vi "ESPControl.vi"(0 "Motion Settings":T1={"No Motion?"=FALSE, "Motion System"=enum."NI 735x", "Motion Bd ID"=1, "Motion Profile"="SMAC1", "# Axis"=1, "Reverse Z axis?"=TRUE, "SMAC Axis"=0, "scan pair"=enum."y-(x) scan", "RT fps"=6.0, "Steps per mm"=[1000, 1000, 1000, 1000], "Motor Parameters"={"velocity ct/s"=[10000.0, 10000.0, 10000.0, 50000.0], "accel ct/s^2"=[50000.0, 50000.0, 50000.0, 200000.0]}, "One Way Scan"=FALSE, "Reverse One Way Scan"=FALSE, "Global Position (mm)"=[], "Plane"=0, "Distance between\nscan lines (um)"=0.0, "Distance between\nscan planes (um)"=0.0, "number of scan planes"=1, "Total steps in line"=0, "Xtra plane\ndistance  (um)"=100, "Xtra planes "=1, "Add Axis"=FALSE, "overshoot cts"=200, "BKPT Shift"=0, "Scan Start Time (ms)"=0, "ESP VISA"="GPIB::1::INSTR", "3rd Axis"=1, "GL Ref Out"=refnum, "Galil Address"=""} {"3rd Axis" items=["x", "y", "z", "w"]; "Xtra planes" min=1; "Xtra plane\ndistance  (um)" min=0; "Distance between\nscan planes (um)" format="%.2f"; "Distance between\nscan lines (um)" format="%.2f"; "SMAC Axis" items=["None"=0, "Axis 1"=1, "Axis 2"=2, "Axis 3"=3, "Axis 4"=4, "Axis 5"=5, "Axis 6"=6, "Axis 7"=7, "Axis 8"=8, "Vector Space 1"=17, "Vector Space 2"=18, "Vector Space 3"=19, "Vector Space 4"=20]; "Motion Bd ID" min=1 max=32 step=1}, 1 "# Axis":u16=2) -> (5 "VISA resource name out":refnum<visa-resource-name>="GPIB::1::INSTR", 6 "Motion Settings Out":T1={"No Motion?"=FALSE, "Motion System"=enum."NI 735x", "Motion Bd ID"=1, "Motion Profile"="SMAC1", "# Axis"=1, "Reverse Z axis?"=TRUE, "SMAC Axis"=0, "scan pair"=enum."y-(x) scan", "RT fps"=6.0, "Steps per mm"=[1000, 1000, 1000, 1000], "Motor Parameters"={"velocity ct/s"=[10000.0, 10000.0, 10000.0, 50000.0], "accel ct/s^2"=[50000.0, 50000.0, 50000.0, 200000.0]}, "One Way Scan"=FALSE, "Reverse One Way Scan"=FALSE, "Global Position (mm)"=[], "Plane"=0, "Distance between\nscan lines (um)"=0.0, "Distance between\nscan planes (um)"=0.0, "number of scan planes"=1, "Total steps in line"=0, "Xtra plane\ndistance  (um)"=100, "Xtra planes "=1, "Add Axis"=FALSE, "overshoot cts"=200, "BKPT Shift"=0, "Scan Start Time (ms)"=0, "ESP VISA"="GPIB::1::INSTR", "3rd Axis"=1, "GL Ref Out"=refnum, "Galil Address"=""} {"3rd Axis" items=["x", "y", "z", "w"]; "Xtra planes" min=1; "Xtra plane\ndistance  (um)" min=0; "Distance between\nscan planes (um)" format="%.2f"; "Distance between\nscan lines (um)" format="%.2f"; "SMAC Axis" items=["None"=0, "Axis 1"=1, "Axis 2"=2, "Axis 3"=3, "Axis 4"=4, "Axis 5"=5, "Axis 6"=6, "Axis 7"=7, "Axis 8"=8, "Vector Space 1"=17, "Vector Space 2"=18, "Vector Space 3"=19, "Vector Space 4"=20]; "Motion Bd ID" min=1 max=32 step=1})   [LabVIEW 2022 SP3]
uses:
  NI_controller/-NI_MotionRoutines/MotionParameters.ctl
  NI_controller/-NI_MotionRoutines/MotionSys.ctl
  -MotionRoutines/ScanAxis.ctl
  -MotionRoutines/3rdAxis.ctl
  <instrlib>/Newport ESP301/Newport ESP301.lvlib
panel:
  in  "Select V&A":bool
  in  "Z Position (mm)":dbl format="%.3f"
  in  "FineMi3":bool
  in  "FinePl3":bool
  in  "Rst3":bool
  in  "Ax3Plus":bool
  in  "Ax3Minus":bool
  in  "Y Position (mm)":dbl format="%.3f"
  in  "FineMi2":bool
  in  "FinePl2":bool
  in  "Rst2":bool
  in  "Ax2Plus":bool
  in  "Ax2Minus":bool
  in  "X Position (mm)":dbl format="%.3f"
  in  "stop":bool
  in  "FineMi1":bool
  in  "FinePl1":bool
  in  "Rst1":bool
  in  "Ax1Plus":bool
  in  "Ax1Minus":bool
  # "© 2010 Riverside Research Institute"
  # "Units are in mm. \"Rst\" zeros the position. Blue circles move 1 cm."
  # "X Axis"
  # "Y Axis"
  # "Z Axis"
  # "1-D and 2-D B scan settings"
  # "1-D and 2-D B scan settings"
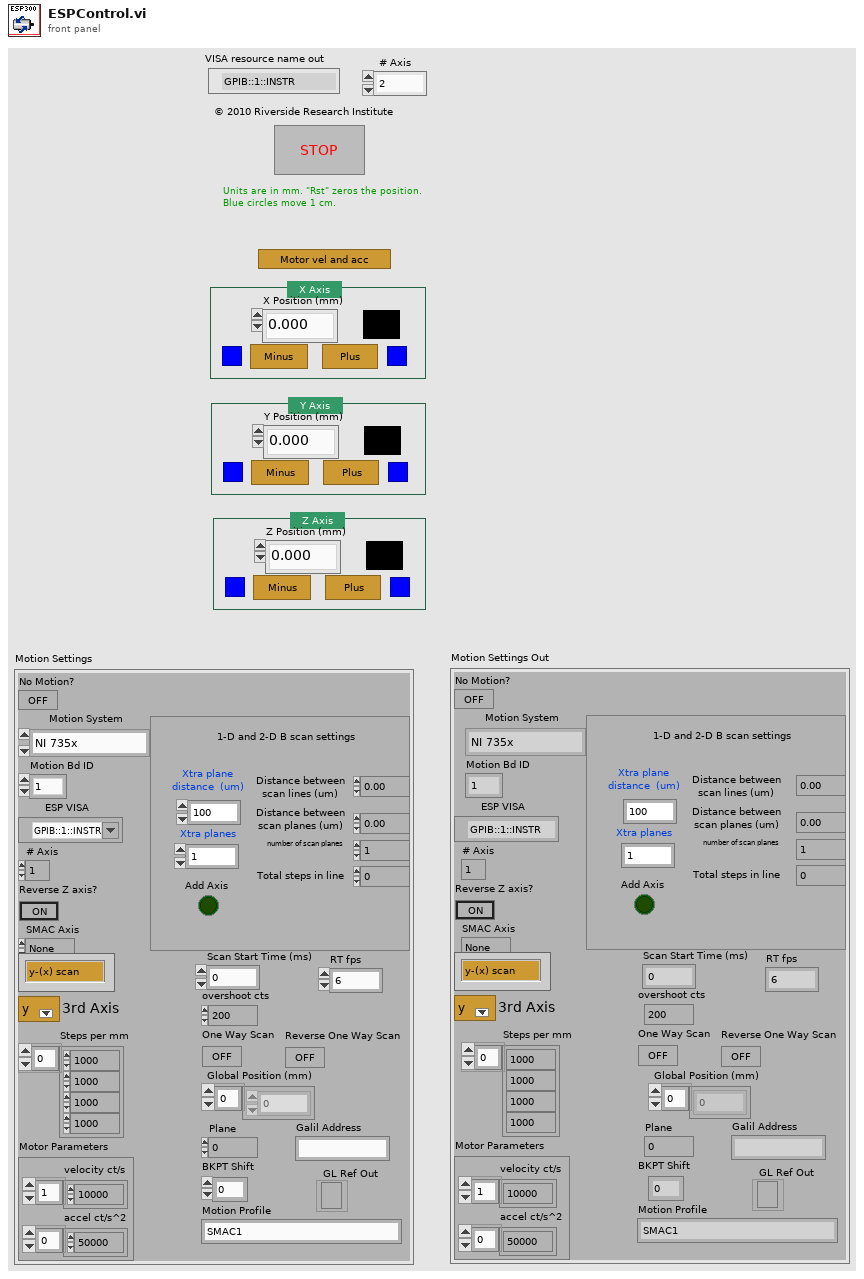
[diagram p1: front panel]
types:
  T1 = typedef "MotionParameters.ctl" = cluster{"No Motion?":bool, "Motion System":T2, "Motion Bd ID":u8, "Motion Profile":string, "# Axis":i8, "Reverse Z axis?":bool, "SMAC Axis":u16, "scan pair":T3, "RT fps":sgl, "Steps per mm":i32[], "Motor Parameters":cluster{"velocity ct/s":dbl[], "accel ct/s^2":dbl[]}, "One Way Scan":bool, "Reverse One Way Scan":bool, "Global Position (mm)":dbl[], "Plane":i32, "Distance between\nscan lines (um)":sgl, "Distance between\nscan planes (um)":sgl, "number of scan planes":i32, "Total steps in line":i32, "Xtra plane\ndistance  (um)":i32, "Xtra planes ":i32, "Add Axis":bool, "overshoot cts":i32, "BKPT Shift":i32, "Scan Start Time (ms)":u32, "ESP VISA":refnum<visa-resource-name>, "3rd Axis":T4, "GL Ref Out":refnum<k7>, "Galil Address":string}
  T2 = typedef "MotionSys.ctl" = enum16{"MM3000", "NI 735x", "Newport ESP", "No Motion Card", "Galil"}
  T3 = typedef "ScanAxis.ctl" = enum16{"y-(x) scan", "x-(y) scan", "z-(x) scan", "z-(y) scan", "y-(z) scan", "x-(z) scan", "w-(x) scan", "w-(y) scan", "w-(z) scan", "x-(w) scan", "y-(w) scan", "z-(w) scan"}
  T4 = typedef "3rdAxis.ctl" = u16
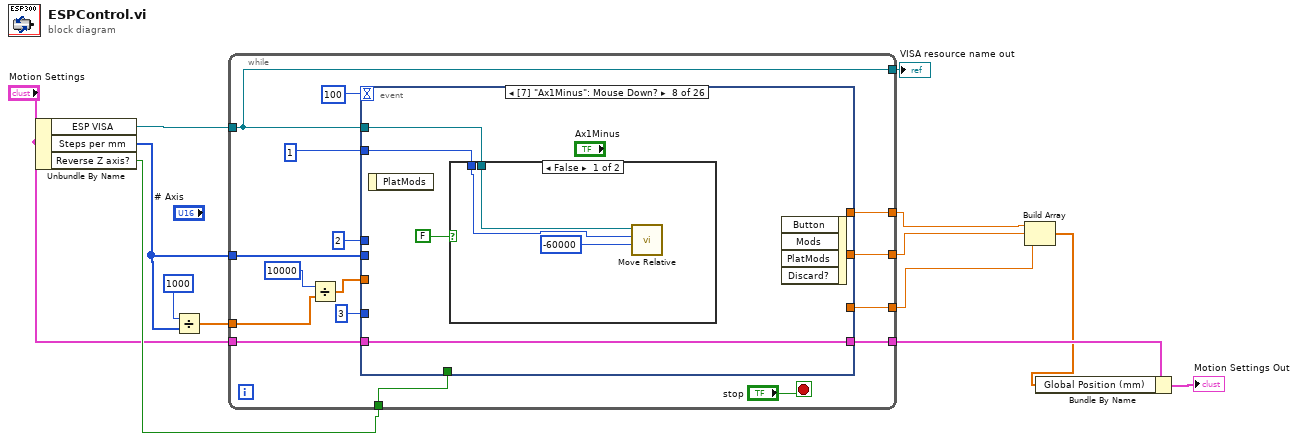
[diagram p0: block diagram]
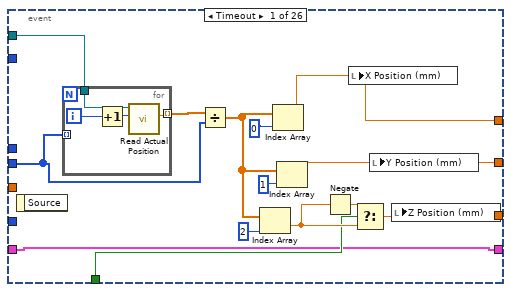
[diagram p2: hidden frame]
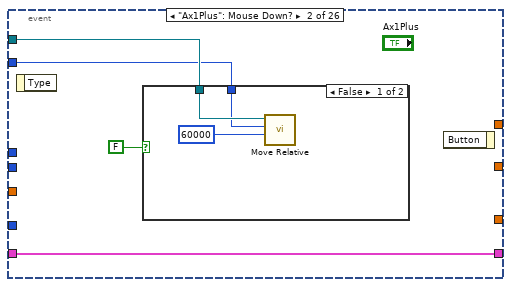
[diagram p3: hidden frame]
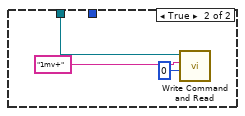
[diagram p4: hidden frame]
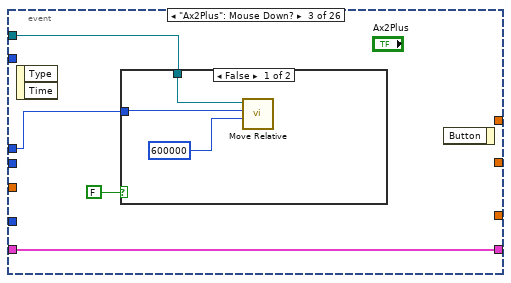
[diagram p5: hidden frame]
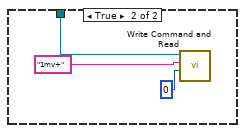
[diagram p6: hidden frame]
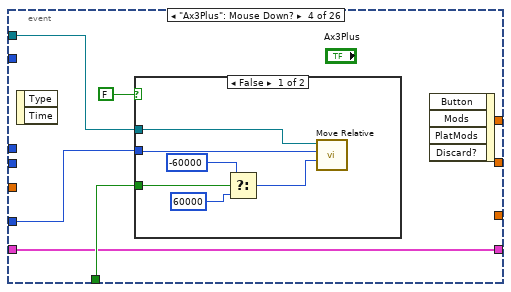
[diagram p7: hidden frame]
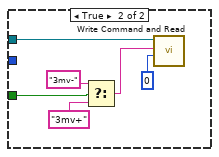
[diagram p8: hidden frame]
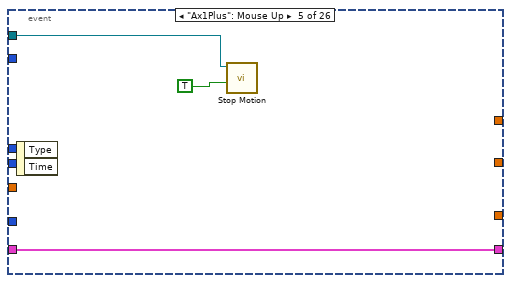
[diagram p9: hidden frame]
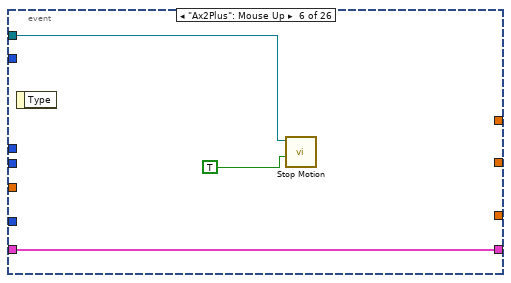
[diagram p10: hidden frame]
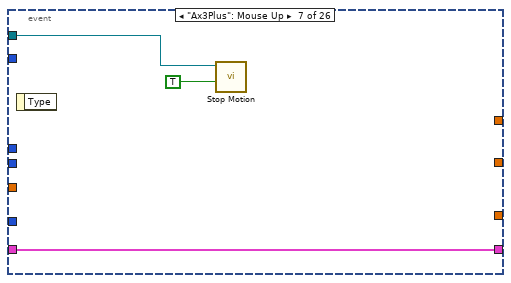
[diagram p11: hidden frame]
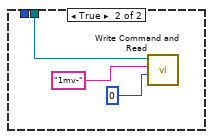
[diagram p12: hidden frame]
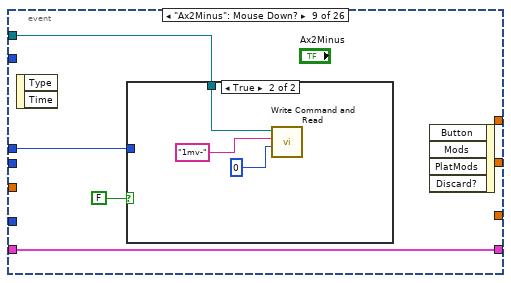
[diagram p13: hidden frame]
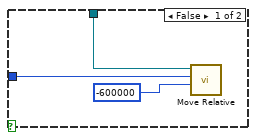
[diagram p14: hidden frame]
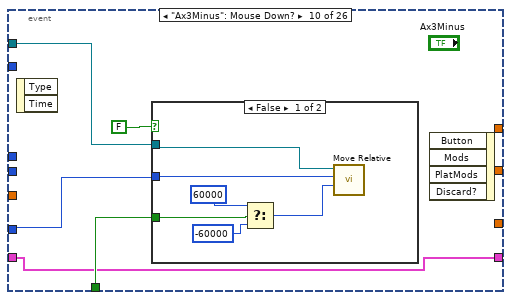
[diagram p15: hidden frame]
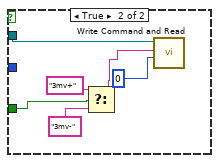
[diagram p16: hidden frame]
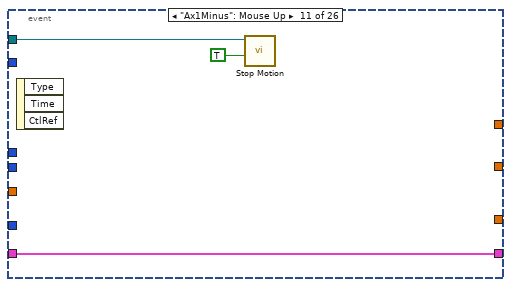
[diagram p17: hidden frame]
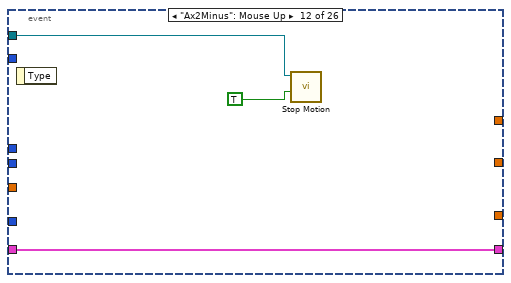
[diagram p18: hidden frame]
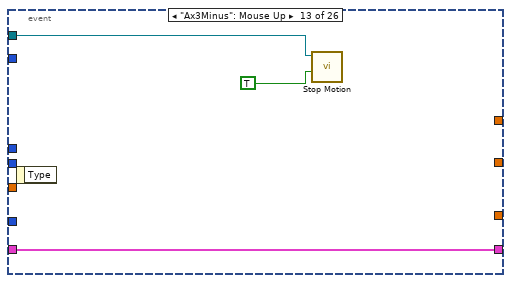
[diagram p19: hidden frame]
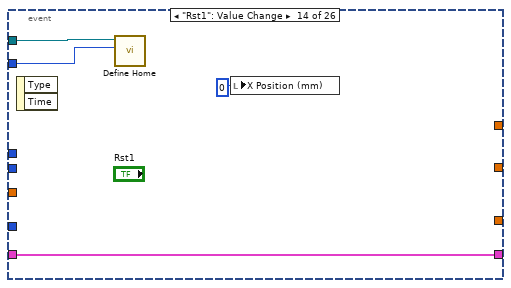
[diagram p20: hidden frame]
diagram:
  n1 = Unbundle By Name("Motion Settings") -> ("ESP VISA"=w6:refnum<visa-resource-name>, "Steps per mm"=w7:i32[], "Reverse Z axis?"=w5:bool)
  n2 = Divide(x=1000, y=w7) -> (x/y=w12:dbl[])
  n3 = while {
    tunnel: w5 -> [w24]
    tunnel: [w28] -> w10
    tunnel: [w27] -> w9
    tunnel: [w26] -> w8
    tunnel: w7 -> [w20]
    tunnel: [w16] -> w13
    tunnel: w12 -> [w17]
    tunnel: w6 -> [w16]
    tunnel: "Motion Settings" -> [w15]
    tunnel: [w14] -> w3
    stop <- "stop" stop-if-true
    n4 = Divide(x=10000, y=w17) -> (x/y=w18:dbl[])
    n5 = event shown="[7] \"Ax1Minus\": Mouse Down?" {
      selector: _ -> [_ _ _ _ _ _ _ _ _ _ _ _ _ _ _ _ _ _ _ _ _ _ _ _ _ _]
      dyn-events: _ -> [_ _ _ _ _ _ _ _ _ _ _ _ _ _ _ _ _ _ _ _ _ _ _ _ _ _]
      timeout: 100 -> [_ _ _ _ _ _ _ _ _ _ _ _ _ _ _ _ _ _ _ _ _ _ _ _ _ _]
      tunnel: 1 -> [_ w49 _ _ _ _ _ w96 _ _ _ _ _ w142 _ _ _ _ _ _ _ _ w214 _ _ _]
      tunnel: w24 -> [w35 _ _ w70 _ _ _ _ _ w116 _ _ _ _ _ _ _ _ w175 _ _ w204 _ _ w228 _]
      tunnel: 2 -> [_ _ w59 _ _ _ _ _ w106 _ _ _ _ _ w146 _ _ _ _ _ _ _ _ w223 _ _]
      tunnel: 3 -> [_ _ _ w71 _ _ _ _ _ w115 _ _ _ _ _ w150 _ _ _ _ _ _ _ _ w233 _]
      tunnel: w18 -> [_ _ _ _ _ _ _ _ _ _ _ _ _ _ _ _ w154 w162 w171 w183 w191 w200 _ _ _ _]
      tunnel: [w38 _ _ _ _ _ _ _ _ _ _ _ _ _ _ _ _ _ _ _ _ _ _ _ _ _] -> w28
      tunnel: [w37 _ _ _ _ _ _ _ _ _ _ _ _ _ _ _ _ _ _ _ _ _ _ _ _ _] -> w27
      tunnel: [w36 _ _ _ _ _ _ _ _ _ _ _ _ _ _ _ _ _ _ _ _ _ _ _ _ _] -> w26
      tunnel: w20 -> [w31 _ _ _ _ _ _ _ _ _ _ _ _ _ _ _ _ _ _ _ _ _ w213 w221 w229 w241]
      tunnel: w16 -> [w34 w51 w60 w69 w87 w90 w93 w97 w107 w118 w133 w136 w139 w141 w145 w149 w156 w165 w174 w185 w194 w203 w215 w222 w234 w242]
      tunnel: w15 -> [w30 w48 w58 w68 w85 w88 w91 w94 w104 w114 w131 w134 w137 w140 w144 w148 w152 w160 w169 w181 w189 w198 w210 w217 w225 w237]
      tunnel: [w30 w48 w58 w68 w85 w88 w91 w94 w104 w114 w131 w134 w137 w140 w144 w148 w152 w160 w169 w181 w189 w198 w210 w217 w225 w236] -> w14
      event Timeout {
        n6 = event-data() -> ()  [unwired: 2 out]
        n7 = for {
          tunnel: [w46] -> w33 mode=indexing
          tunnel: w34 -> [w44]
          tunnel: w31 -> [_] mode=indexing
          i -> [w47]
          n8 = Increment(x=w47) -> (x+1=w45:i32)
          n9 = call <instrlib>:"Read Actual Position.vi"("Axis (1)"=w45, "VISA resource name"=w44) -> ("Position (units)"=w46:dbl)  [unwired: 3 in, 2 out]
        }
        n10 = Divide(x=w33, y=w31) -> (x/y=w32:dbl[])
        n11 = Index Array(array=w32, index=2 ("Axis")) -> (element=w39:dbl)
        n12 = Index Array(array=w32, index=0 ("Index")) -> (element=w38:dbl)
        n13 = Index Array(array=w32, index=1 ("Axis")) -> (element=w37:dbl)
        n14 = Negate(x=w39) -> (-x=w40:dbl)
        n15 = local write "X Position (mm)"(w38) -> ()
        n16 = Select(t=w40, s=w35, f=w39) -> (s? t:f=w36:dbl)
        n17 = local write "Y Position (mm)"(w37) -> ()
        n18 = local write "Z Position (mm)"(w36) -> ()
      }
      event "Ax1Plus": Mouse Down? {
        n19 = event-data() -> ()  [unwired: 2 out]
        n20 = case shown="False" FALSE {
          tunnel: w51 -> [w54 w56]
          tunnel: w49 -> [w53 _]
          frame False {
            n21 = call <instrlib>:"Move Relative.vi"("Position (0 units)"=60000 ("Axis (1)"), "Axis (1)"=w53, "VISA resource name"=w54) -> ()  [unwired: 3 in, 2 out]
          }
          frame True {
            n22 = call <instrlib>:"Write Command and Read.vi"("Bytes to read (100)"=u32 0, "Command"="1mv+", "VISA resource name"=w56) -> ()  [unwired: 4 in, 3 out]
          }
        }
        n23 = event-data() -> ()  [unwired: 2 in, 1 out]
      }
      event "Ax2Plus": Mouse Down? {
        n24 = event-data() -> ()  [unwired: 3 out]
        n25 = case shown="False" FALSE {
          tunnel: w60 -> [w64 w66]
          tunnel: w59 -> [w63 _]
          frame False {
            n26 = call <instrlib>:"Move Relative.vi"("Position (0 units)"=600000 ("Axis (1)"), "Axis (1)"=w63, "VISA resource name"=w64) -> ()  [unwired: 3 in, 2 out]
          }
          frame True {
            n27 = call <instrlib>:"Write Command and Read.vi"("Bytes to read (100)"=u32 0, "Command"="1mv+", "VISA resource name"=w66) -> ()  [unwired: 4 in, 3 out]
          }
        }
        n28 = event-data() -> ()  [unwired: 2 in, 1 out]
      }
      event "Ax3Plus": Mouse Down? {
        n29 = event-data() -> ()  [unwired: 3 out]
        n30 = case shown="False" FALSE {
          tunnel: w69 -> [w78 w84]
          tunnel: w71 -> [w77 _]
          tunnel: w70 -> [w73 w79]
          frame False {
            n31 = Select(t=-60000 ("y"), s=w73, f=60000 ("y")) -> (s? t:f=w74:i32)
            n32 = call <instrlib>:"Move Relative.vi"("Position (0 units)"=w74, "Axis (1)"=w77, "VISA resource name"=w78) -> ()  [unwired: 3 in, 2 out]
          }
          frame True {
            n33 = Select(t="3mv-", s=w79, f="3mv+") -> (s? t:f=w80:string)
            n34 = call <instrlib>:"Write Command and Read.vi"("Bytes to read (100)"=0, "Command"=w80, "VISA resource name"=w84) -> ()  [unwired: 4 in, 3 out]
          }
        }
        n35 = event-data() -> ()  [unwired: 5 in, 1 out]
      }
      event "Ax1Plus": Mouse Up {
        n36 = event-data() -> ()  [unwired: 3 out]
        n37 = call <instrlib>:"Stop Motion.vi"("Stop all axes (F)"=TRUE, "VISA resource name"=w87) -> ()  [unwired: 4 in, 2 out]
      }
      event "Ax2Plus": Mouse Up {
        n38 = event-data() -> ()  [unwired: 2 out]
        n39 = call <instrlib>:"Stop Motion.vi"("Stop all axes (F)"=TRUE, "VISA resource name"=w90) -> ()  [unwired: 4 in, 2 out]
      }
      event "Ax3Plus": Mouse Up {
        n40 = event-data() -> ()  [unwired: 2 out]
        n41 = call <instrlib>:"Stop Motion.vi"("Stop all axes (F)"=TRUE, "VISA resource name"=w93) -> ()  [unwired: 4 in, 2 out]
      }
      event "Ax1Minus": Mouse Down? {
        n42 = event-data() -> ()  [unwired: 2 out]
        n43 = case shown="False" FALSE {
          tunnel: w97 -> [w99 w102]
          tunnel: w96 -> [w98 _]
          frame False {
            n44 = call <instrlib>:"Move Relative.vi"("Position (0 units)"=-60000 ("Axis (1)"), "Axis (1)"=w98, "VISA resource name"=w99) -> ()  [unwired: 3 in, 2 out]
          }
          frame True {
            n45 = call <instrlib>:"Write Command and Read.vi"("Bytes to read (100)"=0, "Command"="1mv-", "VISA resource name"=w102) -> ()  [unwired: 4 in, 3 out]
          }
        }
        n46 = event-data() -> ()  [unwired: 5 in, 1 out]
      }
      event "Ax2Minus": Mouse Down? {
        n47 = event-data() -> ()  [unwired: 3 out]
        n48 = case shown="True" FALSE {
          tunnel: w107 -> [w109 w112]
          tunnel: w106 -> [w108 _]
          frame False {
            n49 = call <instrlib>:"Move Relative.vi"("Position (0 units)"=-600000 ("Axis (1)"), "Axis (1)"=w108, "VISA resource name"=w109) -> ()  [unwired: 3 in, 2 out]
          }
          frame True {
            n50 = call <instrlib>:"Write Command and Read.vi"("Bytes to read (100)"=0, "Command"="1mv-", "VISA resource name"=w112) -> ()  [unwired: 4 in, 3 out]
          }
        }
        n51 = event-data() -> ()  [unwired: 5 in, 1 out]
      }
      event "Ax3Minus": Mouse Down? {
        n52 = event-data() -> ()  [unwired: 3 out]
        n53 = case shown="False" FALSE {
          tunnel: w118 -> [w124 w130]
          tunnel: w115 -> [w123 _]
          tunnel: w116 -> [w119 w125]
          frame False {
            n54 = Select(t=60000 ("y"), s=w119, f=-60000 ("y")) -> (s? t:f=w120:i32)
            n55 = call <instrlib>:"Move Relative.vi"("Position (0 units)"=w120, "Axis (1)"=w123, "VISA resource name"=w124) -> ()  [unwired: 3 in, 2 out]
          }
          frame True {
            n56 = Select(t="3mv+", s=w125, f="3mv-") -> (s? t:f=w126:string)
            n57 = call <instrlib>:"Write Command and Read.vi"("Bytes to read (100)"=0, "Command"=w126, "VISA resource name"=w130) -> ()  [unwired: 4 in, 3 out]
          }
        }
        n58 = event-data() -> ()  [unwired: 5 in, 1 out]
      }
      event "Ax1Minus": Mouse Up {
        n59 = event-data() -> ()  [unwired: 4 out]
        n60 = call <instrlib>:"Stop Motion.vi"("Stop all axes (F)"=TRUE, "VISA resource name"=w133) -> ()  [unwired: 4 in, 2 out]
      }
      event "Ax2Minus": Mouse Up {
        n61 = event-data() -> ()  [unwired: 2 out]
        n62 = call <instrlib>:"Stop Motion.vi"("Stop all axes (F)"=TRUE, "VISA resource name"=w136) -> ()  [unwired: 4 in, 2 out]
      }
      event "Ax3Minus": Mouse Up {
        n63 = event-data() -> ()  [unwired: 2 out]
        n64 = call <instrlib>:"Stop Motion.vi"("Stop all axes (F)"=TRUE, "VISA resource name"=w139) -> ()  [unwired: 4 in, 2 out]
      }
      event "Rst1": Value Change {
        n65 = event-data() -> ()  [unwired: 3 out]
        n66 = call <instrlib>:"Define Home.vi"("Axis (1)"=w142, "VISA resource name"=w141) -> ()  [unwired: 4 in, 2 out]
        n67 = local write "X Position (mm)"(0 ("Primary Reset Position (0)")) -> ()
      }
      event "Rst2": Value Change {
        n68 = event-data() -> ()  [unwired: 2 out]
        n69 = call <instrlib>:"Define Home.vi"("Axis (1)"=w146, "VISA resource name"=w145) -> ()  [unwired: 4 in, 2 out]
        n70 = local write "Y Position (mm)"(0 ("Primary Reset Position (0)")) -> ()
      }
      event "Rst3": Value Change {
        n71 = event-data() -> ()  [unwired: 4 out]
        n72 = call <instrlib>:"Define Home.vi"("Axis (1)"=w150, "VISA resource name"=w149) -> ()  [unwired: 4 in, 2 out]
        n73 = local write "Z Position (mm)"(0 ("Primary Reset Position (0)")) -> ()
      }
      event "FinePl1": Value Change {
        # "# of counts for 1cm"
        n74 = event-data() -> ()  [unwired: 4 out]
        n75 = Index Array(array=w154) -> (element=w153:dbl)  [unwired: 1 in]
        n76 = To Long Integer(number=w153) -> (32bit integer=w157:i32)
        n77 = Format Value(format string="1pr%d", value (0)=w157) -> (output string=w158:string)  [unwired: 1 out]
        n78 = call <instrlib>:"Write Command and Read.vi"("Bytes to read (100)"=0, "Command"=w158, "VISA resource name"=w156) -> ()  [unwired: 4 in, 3 out]
      }
      event "FinePl2": Value Change {
        n79 = event-data() -> ()  [unwired: 2 out]
        n80 = Index Array(array=w162, index=1) -> (element=w161:dbl)
        n81 = To Long Integer(number=w161) -> (32bit integer=w166:i32)
        n82 = Format Value(format string="2pr%d", value (0)=w166) -> (output string=w167:string)  [unwired: 1 out]
        n83 = call <instrlib>:"Write Command and Read.vi"("Bytes to read (100)"=0, "Command"=w167, "VISA resource name"=w165) -> ()  [unwired: 4 in, 3 out]
      }
      event "FinePl3": Value Change {
        n84 = event-data() -> ()  [unwired: 3 out]
        n85 = Index Array(array=w171, index=2) -> (element=w170:dbl)
        n86 = Select(t="3pr-%d", s=w175, f="3pr%d") -> (s? t:f=w176:string)
        n87 = To Long Integer(number=w170) -> (32bit integer=w179:i32)
        n88 = Format Value(format string=w176, value (0)=w179) -> (output string=w180:string)  [unwired: 1 out]
        n89 = call <instrlib>:"Write Command and Read.vi"("Bytes to read (100)"=0, "Command"=w180, "VISA resource name"=w174) -> ()  [unwired: 4 in, 3 out]
      }
      event "FineMi1": Value Change {
        # "# of counts for 1cm"
        n90 = event-data() -> ()  [unwired: 4 out]
        n91 = Index Array(array=w183) -> (element=w182:dbl)  [unwired: 1 in]
        n92 = To Long Integer(number=w182) -> (32bit integer=w186:i32)
        n93 = Format Value(format string="1pr-%d", value (0)=w186) -> (output string=w187:string)  [unwired: 1 out]
        n94 = call <instrlib>:"Write Command and Read.vi"("Bytes to read (100)"=0, "Command"=w187, "VISA resource name"=w185) -> ()  [unwired: 4 in, 3 out]
      }
      event "FineMi2": Value Change {
        n95 = event-data() -> ()  [unwired: 3 out]
        n96 = Index Array(array=w191, index=1) -> (element=w190:dbl)
        n97 = To Long Integer(number=w190) -> (32bit integer=w195:i32)
        n98 = Format Value(format string="2pr-%d", value (0)=w195) -> (output string=w196:string)  [unwired: 1 out]
        n99 = call <instrlib>:"Write Command and Read.vi"("Bytes to read (100)"=0, "Command"=w196, "VISA resource name"=w194) -> ()  [unwired: 4 in, 3 out]
      }
      event "FineMi3": Value Change {
        n100 = event-data() -> ()  [unwired: 2 out]
        n101 = Index Array(array=w200, index=2) -> (element=w199:dbl)
        n102 = Select(t="3pr%d", s=w204, f="3pr-%d") -> (s? t:f=w205:string)
        n103 = To Long Integer(number=w199) -> (32bit integer=w208:i32)
        n104 = Format Value(format string=w205, value (0)=w208) -> (output string=w209:string)  [unwired: 1 out]
        n105 = call <instrlib>:"Write Command and Read.vi"("Bytes to read (100)"=0, "Command"=w209, "VISA resource name"=w203) -> ()  [unwired: 4 in, 3 out]
      }
      event "X Position (mm)": Value Change {
        n106 = event-data() -> ("NewVal"=w216:dbl)  [unwired: 1 out]
        n107 = Index Array(array=w213) -> (element=w212:i32)  [unwired: 1 in]
        n108 = Multiply(x=w216, y=w212) -> (x*y=w211:dbl)
        n109 = call <instrlib>:"Move Absolute.vi"("Position (0 units)"=w211, "Axis (1)"=w214, "VISA resource name"=w215) -> ()  [unwired: 3 in, 2 out]
      }
      event "Y Position (mm)": Value Change {
        n110 = event-data() -> ("NewVal"=w224:dbl)  [unwired: 1 out]
        n111 = Index Array(array=w221, index=1) -> (element=w220:i32)
        n112 = Multiply(x=w220, y=w224) -> (x*y=w218:dbl)
        n113 = call <instrlib>:"Move Absolute.vi"("Position (0 units)"=w218, "Axis (1)"=w223, "VISA resource name"=w222) -> ()  [unwired: 3 in, 2 out]
      }
      event "Z Position (mm)": Value Change {
        n114 = event-data() -> ("NewVal"=w235:dbl)  [unwired: 1 out]
        n115 = Index Array(array=w229, index=2) -> (element=w227:i32)
        n116 = Negate(x=w227) -> (-x=w231:i32)
        n117 = Select(t=w231, s=w228, f=w227) -> (s? t:f=w230:i32)
        n118 = Multiply(x=w235, y=w230) -> (x*y=w226:dbl)
        n119 = call <instrlib>:"Move Absolute.vi"("Position (0 units)"=w226, "Axis (1)"=w233, "VISA resource name"=w234) -> ()  [unwired: 3 in, 2 out]
      }
      event "Select V&A": Value Change {
        n120 = event-data() -> ()  [unwired: 3 out]
        n121 = call "UpdateVandAGlobals.vi"("Motion Settings"=w237) -> ("Motion Settings Out"=w236:T1)  [unwired: 3 in, 1 out]
        n122 = Unbundle By Name(w236) -> ("Motor Parameters.velocity ct/s"=w239:dbl[], "Motor Parameters.accel ct/s^2"=w240:dbl[])
        n123 = for {
          tunnel: w242 -> [w247]
          tunnel: w241 -> [_] mode=indexing
          tunnel: w240 -> [w244] mode=indexing
          tunnel: w239 -> [w243] mode=indexing
          i -> [w249]
          n124 = Increment(x=w249) -> (x+1=w248:i32)
          n125 = call <instrlib>:"Set Acceleration.vi"("Acceleration (0 units/s²)"=w244, "Axis (1)"=w248, "VISA resource name"=w247) -> ("error out"=w251:errorcluster, "VISA resource name out"=w250:refnum<visa-resource-name>)  [unwired: 3 in]
          n126 = call <instrlib>:"Set Deceleration.vi"("error in (no error)"=w251, "Deceleration (0 units/s²)"=w244, "Axis (1)"=w248, "VISA resource name"=w250) -> ("error out"=w245:errorcluster, "VISA resource name out"=w246:refnum<visa-resource-name>)  [unwired: 2 in]
          n127 = call <instrlib>:"Set Velocity.vi"("error in (no error)"=w245, "Axis (1)"=w243, "VISA resource name"=w246) -> ()  [unwired: 3 in, 2 out]
        }
        n128 = local write "Select V&A"(FALSE ("Select V&A")) -> ()
      }
    }
  }
  "VISA resource name out" <- w13
  n129 = Build Array(w10, w9, w8) -> (w2:dbl[])
  n130 = Bundle By Name(cluster=w3, "Global Position (mm)"=w2) -> (→"Motion Settings Out":T1)
